vi "Read Data4DIM.vi"(8 "error in (no error)":errorcluster, 11 "BME_DG_Chnl in":refnum<class "BME_DG_Chnl.lvclass">) -> (0 "error out":errorcluster, 1 "DIMServiceID":i32, 2 "DIMData":string, 3 "BME_DG_Chnl out":refnum<class "BME_DG_Chnl.lvclass">)   [LabVIEW 2009, in "POLARIS BME DG.lvlib" / "BME_DG_Chnl.lvclass"]
uses:
  BME_DG_Chnl.lvclass
  BME_DG_Chnl.lvclass/BME_DG_Chnl.ctl
panel:
  in  "x":dbl
  in  "Numeric":i32=123
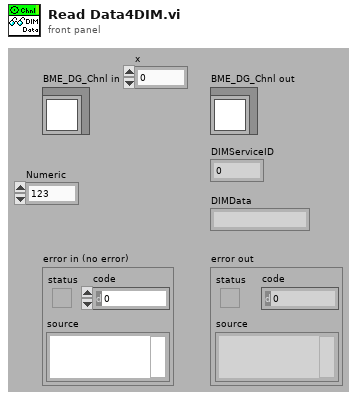
[diagram p1: front panel]
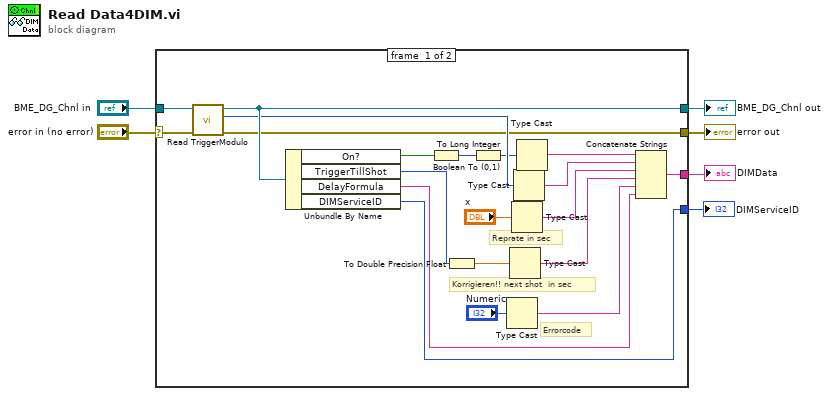
[diagram p0: block diagram]
diagram:
  n1 = case shown="No Error" "error in (no error)" {
    selector: "error in (no error)" -> [w15 w28]
    tunnel: [w14 w28] -> w5
    tunnel: [w24 w27] -> w3
    tunnel: "BME_DG_Chnl in" -> [w25 w27]
    tunnel: [w13 _] -> w2
    tunnel: [w11 _] -> w1
    frame #0 {
      # "Errorcode"
      # "Korrigieren!! next shot  in sec"
      # "Reprate in sec"
      n2 = call-dynamic "Read TriggerModulo.vi"("error in (no error)"=w15, "BME_DG_Chnl in"=w25) -> ("error out"=w14:errorcluster, "TriggerModulo"=w23:i32, "BME_DG_Chnl out"=w24:refnum<class "BME_DG_Chnl.lvclass">)  [unwired: 7 in]
      n3 = Unbundle By Name(w24) -> ("On?"=w26:bool, "TriggerTillShot"=w21:i32, "DelayFormula"=w7:string, "DIMServiceID"=w11:i32)
      n4 = Boolean To (0,1)(Boolean=w26) -> (0, 1=w10:i16)
      n5 = To Double Precision Float(number=w21) -> (double precision float=w12:dbl)
      n6 = To Long Integer(number=w10) -> (32bit integer=w9:i32)
      n7 = Type Cast(x="Numeric") -> (*(type *) &x=w8:string)  [unwired: 1 in]
      n8 = Type Cast(x=w12) -> (*(type *) &x=w16:string)  [unwired: 1 in]
      n9 = Type Cast(x="x") -> (*(type *) &x=w17:string)  [unwired: 1 in]
      n10 = Type Cast(x=w23) -> (*(type *) &x=w18:string)  [unwired: 1 in]
      n11 = Type Cast(x=w9) -> (*(type *) &x=w19:string)  [unwired: 1 in]
      n12 = Concatenate Strings(w19, w18, w17, w16, w8, w7) -> (w13:string)
    }
    frame #1 {
    }
  }
  "error out" <- w5
  "BME_DG_Chnl out" <- w3
  "DIMData" <- w2
  "DIMServiceID" <- w1
